vi "CPP-ZeroMaintenance.vi"(2 "Previous Scan Value":dbl, 3 "Ch Description":T2={"Ch Name"="Tunnel3:Pressures:", "Type"="", "Function"=enum."Analogue Input", "Ch State"=enum."On", "Calibration type"="", "A"=30.0, "B"=10.0, "C"=0.0, "D"=0.0, "Comments"="", "Address"={"Main"=0, "Ch."=0, "Sub"=0, "Port Name"=""}, "String"="", "Duty"=65535} {"Duty" format="%016b"; "D" format="%#_5g"; "C" format="%#_5g"; "B" format="%#_5g"; "A" format="%#_5g"}) -> (0 "Time Elapsed since zero (min)":dbl format="%#.2f", 1 "HelpText":string)   [LabVIEW 2022 SP3]
doc: "This VI performs the Auto Zeroing routine. All of the information for a given Rig should be included in the Channel Description for this to work correctly. The Channel name is not terribly important, but the assumed convention is < Rig Name >:Pressures:\n\nA := Seconds to Monitor is the interval used to determine whether the tunnel has been off long enough\nB := Seconds to Average is the averaging interval for recording zeroes\nC := timestamp of most recent Zero\nD := timestamp of previous Zero\n\nThe String element should be a semi-colon-separated array of ADAM Chs. The first Ch in the array should be the Listener Ch which is compared with the Threshold to determine if the tunnel is OFF. The remaining array of ADAM Chs should be all of the Pressure Chs that are to be auto-zeroed."
uses:
  ADAM Client/Sub VIs/ADAM Controls/Ch_description_ADAM.ctl
  ADAM Client/Sub VIs/ADAM Controls/Module_type_ADAM.ctl
  ADAM Client/Sub VIs/ADAM Controls/Function_ADAM.ctl
  ADAM Client/Sub VIs/ADAM Controls/Channel_State.ctl
  ADAM Client/Sub VIs/ADAM Controls/Calib_type_ADAM.ctl
  ADAM Client/Sub VIs/ADAM Controls/Address.ctl
panel:
  in  "Tab Control":T1(tab)
  out "Listener Threshold":dbl
  out "Fresh Data Available?":bool
  out "Do Zeroes?":bool
  out "Below Threshold?":bool
  out "Listening Ch":string[](array[string])
  out "Pressure Chs":string[](array[string])
  out "Listening Value":dbl=0.2694398123338766
  out "current time":timestamp=timestamp(3521053420.076362 s since 1904-01-01)
  out "Current Time (sec)":dbl=3521053420.076362 format="%#.0f"
  out "LastZeroedSS":dbl=3521053410.165856 format="%#.0f"
  in  "Throwback (s)":dbl=10.0 format="%#_13g"
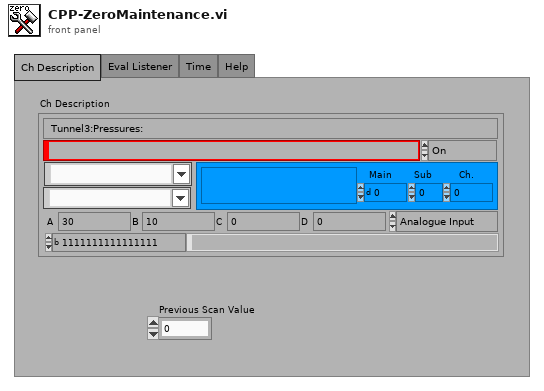
[diagram p1: front panel]
types:
  T1 = enum32{"Ch Description", "Eval Listener", "Time", "Help"}
  T2 = typedef "Ch_description_ADAM.ctl" = cluster{"Ch Name":string, "Type":T3, "Function":T4, "Ch State":T5, "Calibration type":T6, "A":dbl, "B":dbl, "C":dbl, "D":dbl, "Comments":string, "Address":T7, "String":string, "Duty":u16}
  T3 = typedef "Module_type_ADAM.ctl" = string
  T4 = typedef "Function_ADAM.ctl" = enum16{"Analogue Input", "Digital Input", "Event counter", "Event rate", "Analogue Output", "Digital Output", "Relay Output"}
  T5 = typedef "Channel_State.ctl" = enum16{"On", "Off", "Always On", "Always Off"}
  T6 = typedef "Calib_type_ADAM.ctl" = string
  T7 = typedef "Address.ctl" = cluster{"Main":i32, "Ch.":i32, "Sub":i32, "Port Name":string}
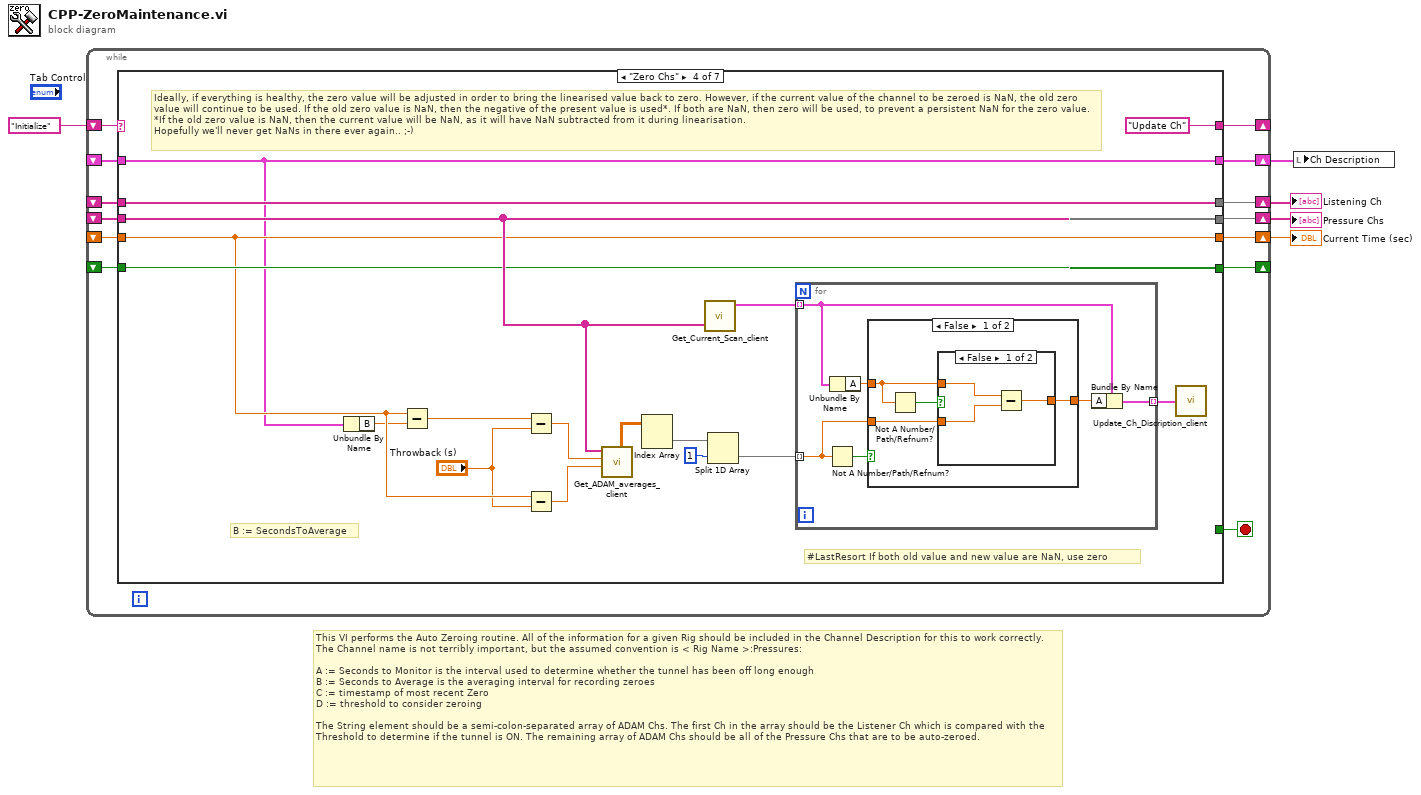
[diagram p0: block diagram]
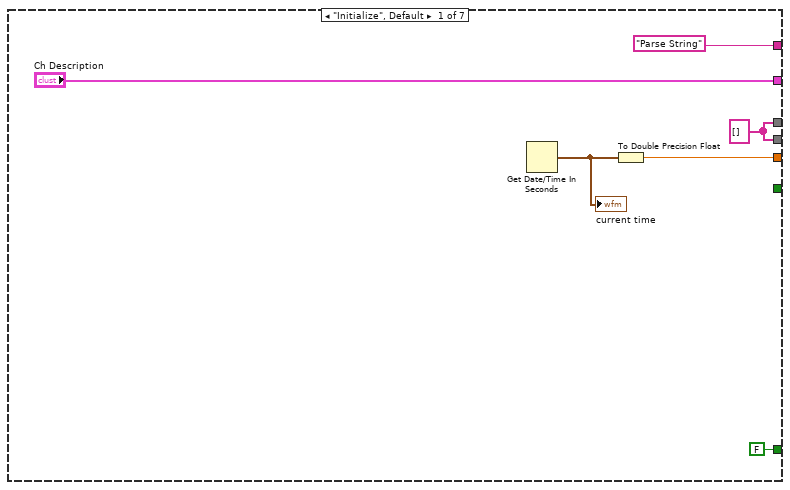
[diagram p2: hidden frame]
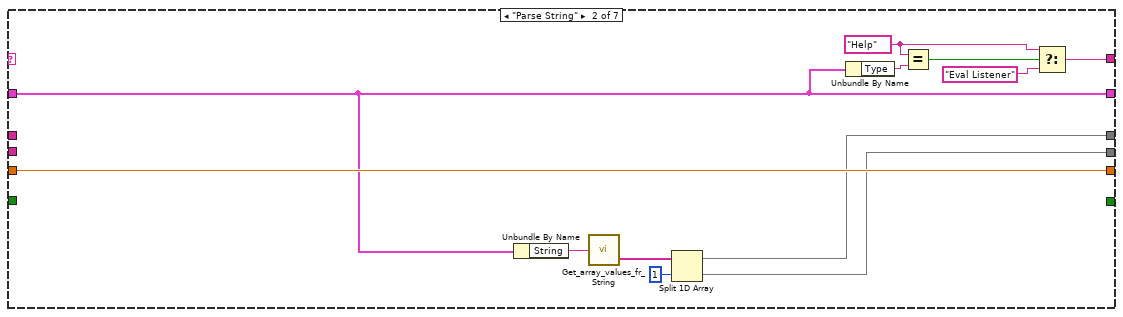
[diagram p3: hidden frame]
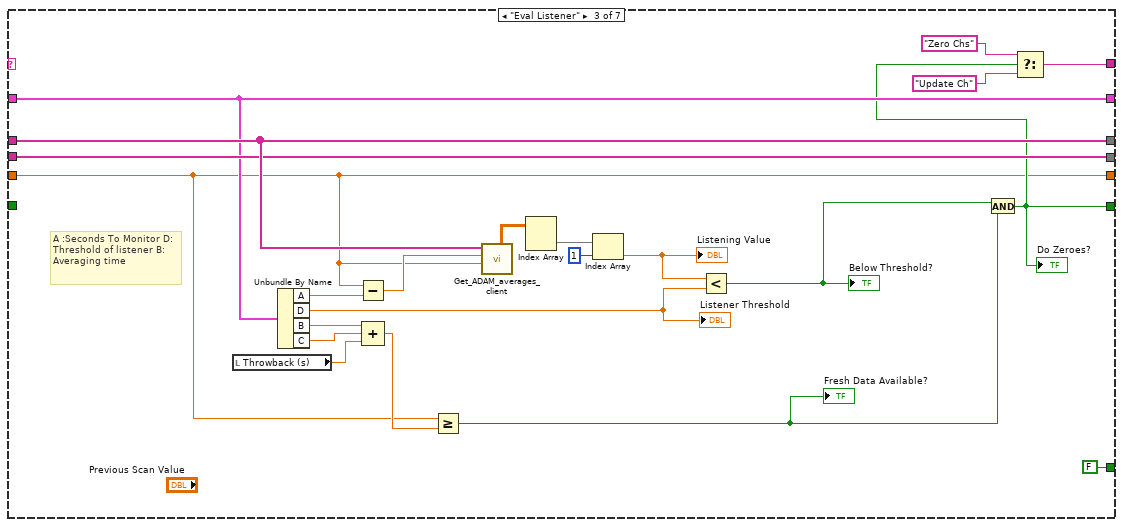
[diagram p4: hidden frame]
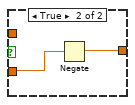
[diagram p5: hidden frame]
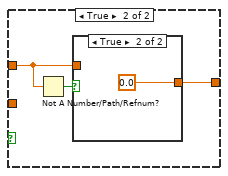
[diagram p6: hidden frame]
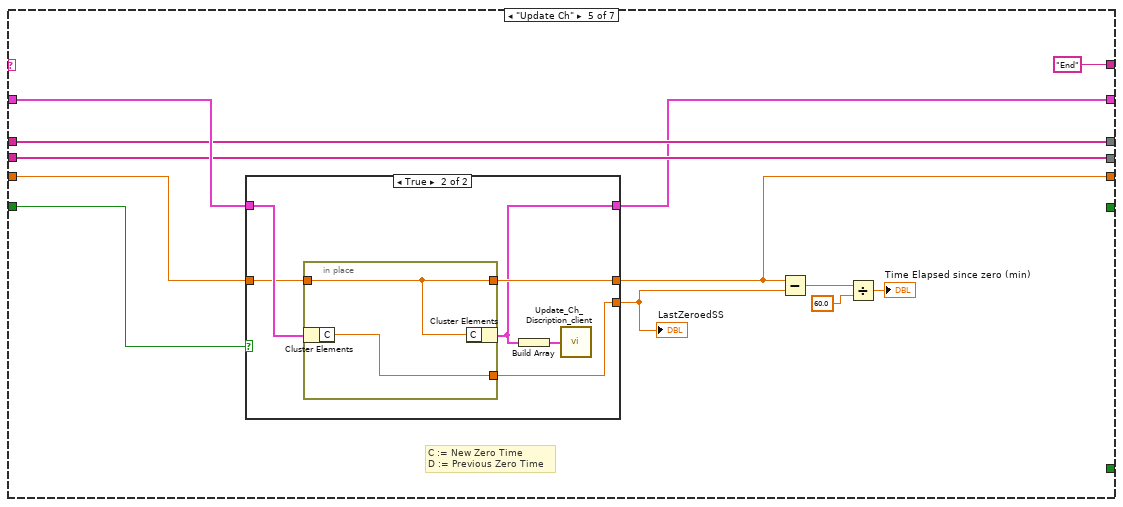
[diagram p8: hidden frame]
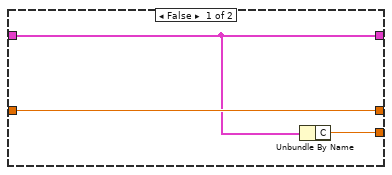
[diagram p9: hidden frame]
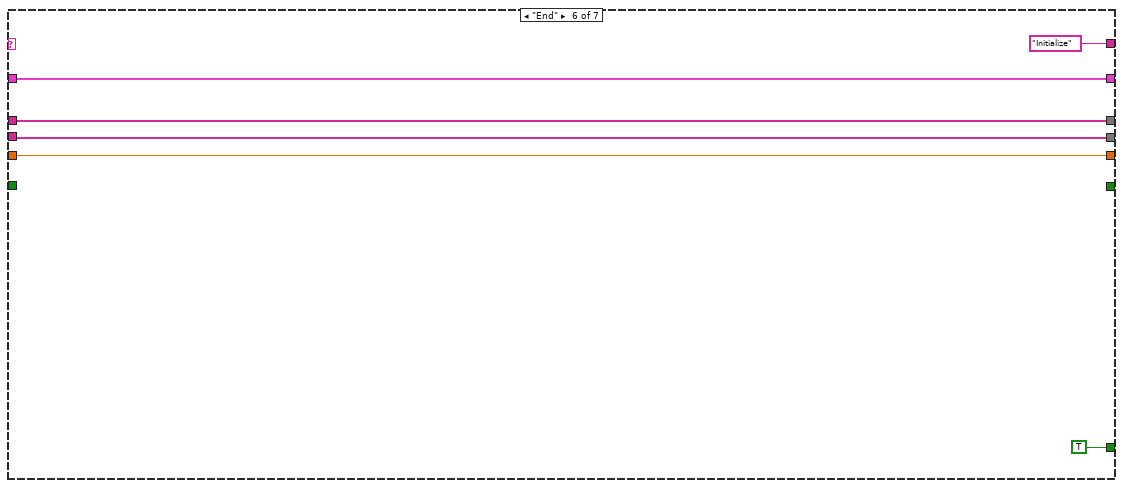
[diagram p10: hidden frame]
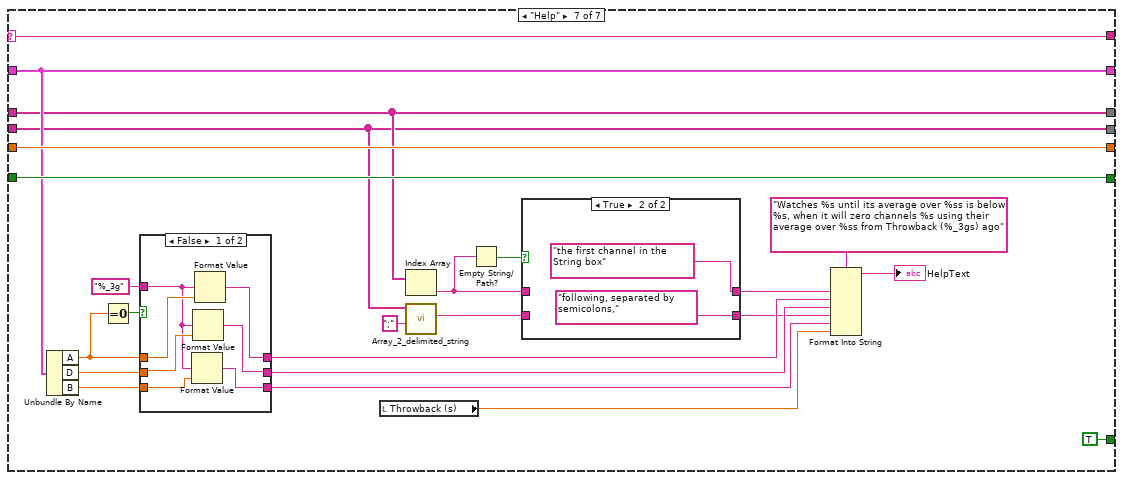
[diagram p11: hidden frame]
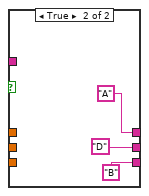
[diagram p13: hidden frame]
diagram:
  # "This VI performs the Auto Zeroing routine. All of the information for a given Rig should be included in the Channel Description for this to work correctly. The Channel name is not terribly important, but the assumed convention is < Rig Name >:Pressures:\n\nA := Seconds to Monitor is the interval used to determine whether the tunnel has been off long enough\nB := Seconds to Average is the averaging interval for recording zeroes\nC := timestamp of most recent Zero\nD := threshold to consider zeroing\n\nThe String element should be a semi-colon-separated array of ADAM Chs. The first Ch in the array should be the Listener Ch which is compared with the Threshold to determine if the tunnel is ON. The remaining array of ADAM Chs should be all of the Pressure Chs that are to be auto-zeroed."
  n1 = while {
    shift-right: [w17] -> _
    shift-left: "Initialize" -> [w18]
    shift-right: [w15] -> w1
    shift-left: _ -> [w16]
    shift-right: [w14] -> w3
    shift-left: _ -> [w13]
    shift-right: [w12] -> w2
    shift-left: _ -> [w11]
    shift-right: [w10] -> w4
    shift-left: _ -> [w8]
    shift-right: [w7] -> _
    shift-left: _ -> [w6]
    stop <- w9 stop-if-true
    n2 = case shown="\"Zero Chs\"" w18 {
      selector: w18 -> [_ _ _ _ _ _ w148]
      tunnel: ["Parse String" w27 w48 "Update Ch" "End" "Initialize" w148] -> w17
      tunnel: w16 -> [_ w26 w53 w70 w107 w123 w144]
      tunnel: ["Ch Description" w26 w53 w70 w97 w123 w144] -> w15
      tunnel: [w22 w32 w55 w74 w99 w121 w143] -> w14
      tunnel: w13 -> [_ _ w55 w74 w99 w121 w143]
      tunnel: [w22 w31 w54 w75 w98 w120 w139] -> w12
      tunnel: w11 -> [_ _ w54 w75 w98 w120 w139]
      tunnel: [w23 w35 w39 w71 w101 w119 w147] -> w10
      tunnel: [FALSE _ FALSE _ _ TRUE TRUE] -> w9
      tunnel: w8 -> [_ w35 w39 w71 w105 w119 w147]
      tunnel: [_ _ w42 w73 _ _ w146] -> w7
      tunnel: w6 -> [_ _ _ w73 w106 _ w146]
      frame "Initialize", Default {
        w22 = string[] []
        n3 = Get Date/Time In Seconds() -> (seconds since 1Jan1904=w24:timestamp)
        "current time" <- w24
        n4 = To Double Precision Float(number=w24) -> (double precision float=w23:dbl)
      }
      frame "Parse String" {
        w28 = T3 "Help" ("Type")
        n5 = Unbundle By Name(w26) -> ("String"=w36:string)
        n6 = call "Get_array_values_fr_String.vi"("String Value"=w36) -> ("String array"=w34:string[])  [unwired: 1 out]
        n7 = Split 1D Array(array=w34, index=1) -> (first subarray=w32:string[], second subarray=w31:string[])
        n8 = Unbundle By Name(w26) -> ("Type"=w25:T3)
        n9 = Equal?(x=w28, y=w25) -> (x = y?=w29:bool)
        n10 = Select(t=w28, s=w29, f="Eval Listener") -> (s? t:f=w27:T3)
      }
      frame "Eval Listener" {
        # "A :Seconds To Monitor D: Threshold of listener B: Averaging time"
        n11 = local read "Throwback (s)"() -> (w37:dbl)
        n12 = Unbundle By Name(w53) -> ("A"=w52:dbl, "D"=w40:dbl, "B"=w41:dbl, "C"=w38:dbl)
        "Listener Threshold" <- w40
        n13 = Subtract(x=w39, y=w52) -> (x-y=w56:dbl)
        n14 = Compound Arithmetic op=ADD(w41, w38, w37) -> (w44:dbl)
        n15 = Greater Or Equal?(x=w39, y=w44) -> (x >= y?=w45:bool)
        "Fresh Data Available?" <- w45
        n16 = call "Get_ADAM_averages_client.vi"("End time"=w39, "Start time"=w56, "ADAM Ch Names"=w55) -> ("DBL values"=w58:dbl[][])  [unwired: 4 in, 4 out]
        n17 = Index Array(array=w58) -> (element=w57:dbl[])  [unwired: 2 in]
        n18 = Index Array(array=w57, index=1) -> (element=w43:dbl)
        "Listening Value" <- w43
        n19 = Less?(x=w43, y=w40) -> (x < y?=w46:bool)
        "Below Threshold?" <- w46
        n20 = And(x=w46, y=w45) -> (x .and. y?=w42:bool)
        "Do Zeroes?" <- w42
        n21 = Select(t="Zero Chs", s=w42, f="Update Ch") -> (s? t:f=w48:string)
      }
      frame "Zero Chs" {
        # "Ideally, if everything is healthy, the zero value will be adjusted in order to bring the linearised value back to zero. However, if the current value of the channel to be zeroed is NaN, the old zero value will continue to be used. If the old zero value is NaN, then the negative of the present value is used*. If both are NaN, then zero will be used, to prevent a persistent NaN for the zero value. *If the old zero value is NaN, then the current value will be NaN, as it will have NaN subtracted from it during linearisation.\nHopefully we'll never get NaNs in there ever again.. ;-)"
        # "#LastResort If both old value and new value are NaN, use zero"
        # "B := SecondsToAverage"
        n22 = Unbundle By Name(w70) -> ("B"=w69:dbl)
        n23 = Subtract(x=w71, y=w69) -> (x-y=w65:dbl)
        n24 = Subtract(x=w65, y="Throwback (s)") -> (x-y=w66:dbl)
        n25 = Subtract(x=w71, y="Throwback (s)") -> (x-y=w67:dbl)
        n26 = call "Get_ADAM_averages_client.vi"("End time"=w67, "Start time"=w66, "ADAM Ch Names"=w75) -> ("DBL values"=w60:dbl[][])  [unwired: 4 in, 4 out]
        n27 = Index Array(array=w60) -> (element=w61:dbl[])  [unwired: 2 in]
        n28 = call "Get_Current_Scan_client.vi"("multipleChannels"=w75) -> ("Ch Description Array"=w59:T2[])  [unwired: 1 in, 3 out]
        n29 = Split 1D Array(array=w61, index=1) -> (second subarray=w62:dbl[])  [unwired: 1 out]
        n30 = for {
          tunnel: w59 -> [w80] mode=indexing
          tunnel: w62 -> [w76] mode=indexing
          tunnel: [w78] -> w64 mode=indexing
          n31 = Not A Number/Path/Refnum?(number/path/refnum=w76) -> (NaN/Path/Refnum?=w77:bool)
          n32 = Unbundle By Name(w80) -> ("A"=w81:dbl)
          n33 = case shown="False" w77 {
            tunnel: w81 -> [w82 w91]
            tunnel: w76 -> [w85 _]
            tunnel: [w84 w92] -> w79
            frame False {
              n34 = Not A Number/Path/Refnum?(number/path/refnum=w82) -> (NaN/Path/Refnum?=w83:bool)
              n35 = case shown="False" w83 {
                tunnel: w82 -> [w88 _]
                tunnel: w85 -> [w87 w89]
                tunnel: [w86 w90] -> w84
                frame False {
                  n36 = Subtract(x=w88, y=w87) -> (x-y=w86:dbl)
                }
                frame True {
                  n37 = Negate(x=w89) -> (-x=w90:dbl)
                }
              }
            }
            frame True {
              n38 = Not A Number/Path/Refnum?(number/path/refnum=w91) -> (NaN/Path/Refnum?=w93:bool)
              n39 = case shown="True" w93 {
                tunnel: [w94 0.0 ("A")] -> w92
                tunnel: w91 -> [w94 _]
                frame False {
                }
                frame True {
                }
              }
            }
          }
          n40 = Bundle By Name(cluster=w80, "A"=w79) -> (w78:T2)
        }
        n41 = call "Update_Ch_Discription_client.vi"("Channels to update In"=w64) -> ()  [unwired: 1 out]
      }
      frame "Update Ch" {
        # "C := New Zero Time\nD := Previous Zero Time"
        n42 = case shown="True" w106 {
          tunnel: w107 -> [w109 w116]
          tunnel: w105 -> [w110 w115]
          tunnel: [w110 w112] -> w101
          tunnel: [w108 w113] -> w96
          tunnel: [w109 w111] -> w97
          frame False {
            n43 = Unbundle By Name(w109) -> ("C"=w108:dbl)
          }
          frame True {
            n44 = in-place {
              in-place-border: w115 -> [w118]
              in-place-border: [w118] -> w112
              in-place-border: [w117] -> w113
              n45 = in-place-cluster #1(w116) -> ("C"=w117:dbl)
              n46 = in-place-cluster #1("C"=w118) -> (w111:T2)
            }
            n47 = Build Array(w111) -> (w114:T2[])
            n48 = call "Update_Ch_Discription_client.vi"("Channels to update In"=w114) -> ()  [unwired: 1 out]
          }
        }
        "LastZeroedSS" <- w96
        n49 = Subtract(x=w101, y=w96) -> (x-y=w102:dbl)
        n50 = Divide(x=w102, y=60.0) -> (x/y=→"Time Elapsed since zero (min)":dbl)
      }
      frame "End" {
      }
      frame "Help" {
        n51 = Unbundle By Name(w144) -> ("A"=w135:dbl, "D"=w133:dbl, "B"=w131:dbl)
        n52 = Equal To 0?(x=w135) -> (x = 0?=w136:bool)
        n53 = case shown="False" w136 {
          tunnel: [w159 "A"] -> w137
          tunnel: w135 -> [w158 _]
          tunnel: [w156 "D"] -> w134
          tunnel: w133 -> [w157 _]
          tunnel: [w154 "B"] -> w132
          tunnel: w131 -> [w155 _]
          tunnel: "%_3g" ("format string") -> [w153 _]
          frame False {
            n54 = Format Value(format string=w153, value (0)=w155) -> (output string=w154:string)  [unwired: 1 in]
            n55 = Format Value(format string=w153, value (0)=w157) -> (output string=w156:string)  [unwired: 1 in]
            n56 = Format Value(format string=w153, value (0)=w158) -> (output string=w159:string)  [unwired: 1 in]
          }
          frame True {
          }
        }
        n57 = local read "Throwback (s)"() -> (w138:dbl)
        n58 = Index Array(array=w143) -> (element=w128:string)  [unwired: 1 in]
        n59 = call "Array_2_delimited_string.vi"("delimiter (Tab)"=";", "Array of Strings"=w139) -> ("delimited string"=w126:string)  [unwired: 9 in]
        n60 = Empty String/Path?(string/path=w128) -> (empty?=w125:bool)
        n61 = case shown="True" w125 {
          tunnel: [w150 "the first channel in the String box"] -> w129
          tunnel: w128 -> [w150 _]
          tunnel: [w149 "following, separated by semicolons," ("delimited string")] -> w127
          tunnel: w126 -> [w149 _]
          frame False {
          }
          frame True {
          }
        }
        n62 = Format Into String(format string="Watches %s until its average over %ss is below  %s, when it will zero channels %s using their average over %ss from Throwback (%_3gs) ago", w129, w137, w134, w127, w132, w138) -> (resulting string=→"HelpText":string)  [unwired: 2 in, 1 out]
      }
    }
  }
  "Current Time (sec)" <- w4
  "Listening Ch" <- w3
  "Pressure Chs" <- w2
  n63 = local write "Ch Description"(w1) -> ()
